vi "Get Routes.vi"(8 "error in (no error)":errorcluster, 11 "Mux in":refnum<class "Mux.lvclass">) -> (0 "error out":errorcluster, 2 "Routes":i32[](array[numeric]), 3 "Mux out":refnum<class "Mux.lvclass">)   [LabVIEW 2022 SP3, in "VideoMux.lvlib" / "Mux.lvclass"]
uses:
  Mux.lvclass
  Mux.lvclass/Mux.ctl
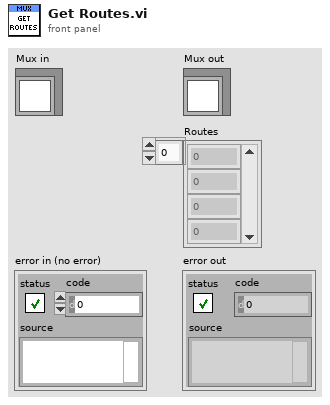
[diagram p1: front panel]
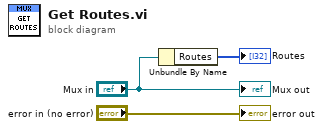
[diagram p0: block diagram]
diagram:
  n1 = Unbundle By Name("Mux in") -> ("Routes"=→"Routes":i32[])
  "error out" <- "error in (no error)"
  "Mux out" <- "Mux in"
